vi "Write Observer Array.vi"(8 "error in (no error)":errorcluster, 10 "Observer Array":refnum<class "Message Enqueuer.lvclass">[](array[class]), 11 "Subject in":refnum<class "Subject.lvclass">) -> (0 "error out":errorcluster, 3 "Subject out":refnum<class "Subject.lvclass">)   [LabVIEW 2013, in "Observer Pattern Actor Interface.lvlib" / "Subject.lvclass"]
uses:
  Subject.lvclass
  <vilib>/ActorFramework/Message Enqueuer/Message Enqueuer.lvclass
  Subject.lvclass/Subject.ctl
  Global 2.vi
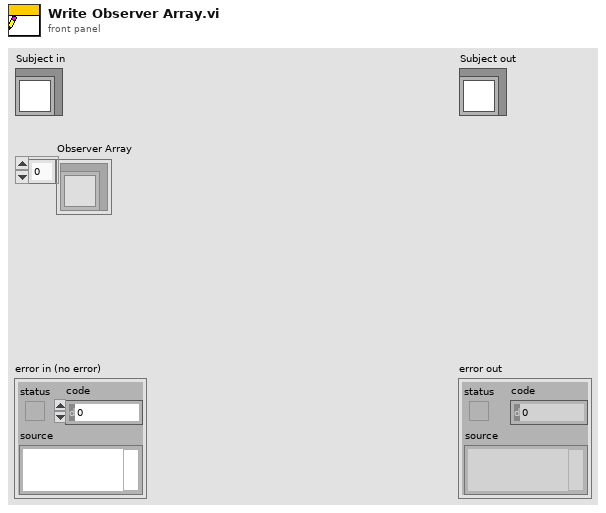
[diagram p1: front panel]
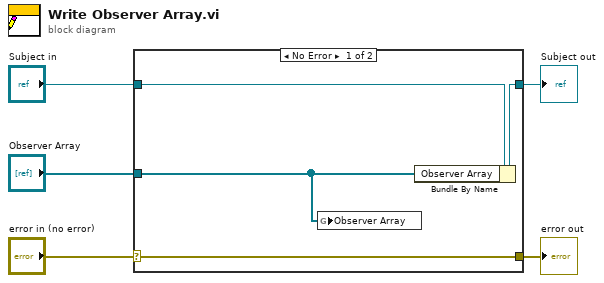
[diagram p0: block diagram]
diagram:
  n1 = case shown="No Error" "error in (no error)" {
    selector: "error in (no error)" -> [w9 w10]
    tunnel: [w9 w10] -> w4
    tunnel: [w7 w11] -> w2
    tunnel: "Subject in" -> [w8 w11]
    tunnel: "Observer Array" -> [w6 _]
    frame No Error {
      n2 = global write "Global 2.vi" "Observer Array"(w6) -> ()
      n3 = Bundle By Name(cluster=w8, "Observer Array"=w6) -> (w7:refnum<class "Subject.lvclass">)
    }
    frame Error {
    }
  }
  "error out" <- w4
  "Subject out" <- w2
